vi "Main.vi"(11 "Module Admin":refnum<class "Delacor_lib_QMH_Module Admin.lvclass">) -> ()   [LabVIEW 2016, in "Impedance Acquisition.lvlib"]
doc: "This template is based off of the Queued Message Handler design pattern and the Queued Message Handler project template that ships with LabVIEW.\n\nThe main difference is that the queue is private to this module and communication between modules is performed via Broadcast and Request events.\n\nRequest events are wrapped in public API methods and are handled in the Event Handling Loop (EHL) of this VI. Any module can register for Broadcast events sent by this module. The EHL generates messages based on user interface actions.\n\nThe Message Handling Loop (MHL) processes messages generated by the EHL, or by other messages. The messages are string values, so new messages can be added easily to the Message Cases case structure in the MHL. Each message cluster can also provide an optional value for Message Data, which is a variant that can be converted to whatever message-specific data is required.\n_____\nBased on DQMH Project Template 6.1.0.94."
uses:
  Impedance Acquisition.lvlib
  <vilib>/Delacor/Delacor QMH/Libraries/Message Queue_class/Delacor_lib_QMH_Message Queue.lvclass
  Module Data--cluster.ctl
  <vilib>/Utility/miscctls.llb/LVPointTypeDef.ctl
  <vilib>/Utility/error.llb/Error Cluster From Error Code.vi
  <vilib>/ErrorRing/Error Ring.xnode
  <vilib>/Delacor/Delacor QMH/Libraries/Message Queue_class/Delacor_lib_QMH_Enqueue Message (Single).vi
  Stop Argument--cluster.ctl
  <vilib>/Delacor/Delacor QMH/Libraries/Module Admin_class/Delacor_lib_QMH_Module Admin.lvclass
  Settings Editor/Settings Editor.lvlib
  Acquisition/Reg_Map.ctl
  Acquisition/Acquisition.lvlib
  Acquisition/WiBCI16T_Status.ctl
  Acquisition/WiBCI16T_Data.ctl
  Start IMP Acq Argument--cluster.ctl
  Start GND LOOP Imp Argument--cluster.ctl
  Stop Imp Acq Argument--cluster.ctl
panel:
  out "error out":errorcluster
  out "Status":string
  in  "Simulate MHL Error":bool
  in  "Simulate EHL Error":bool
  # "Other QMH Modules communicate with this Module via its Public API (wrappers for its Request Events).\n\nThis Module communicates with other Modules via its Broadcast Events.\nAny module that wants to get these messages, just registers for this module's Broadcast events."
  # "This template is for the Delacor Modified Queued Message Handler design pattern.\n\nSee the block diagram for more information on how to use this template."
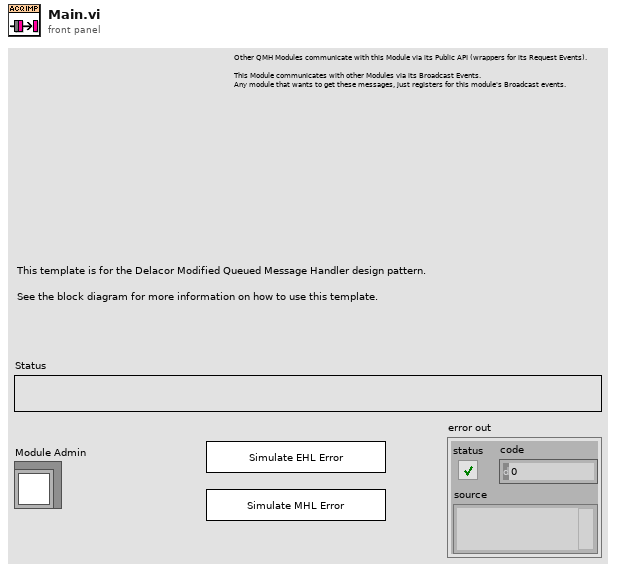
[diagram p1: front panel]
types:
  T1 = typedef "Impedance Acquisition.lvlib/Request Events--cluster.ctl" = cluster{"Stop Module":refnum<user-event>, "Show Panel":refnum<user-event>, "Hide Panel":refnum<user-event>, "Get Module Execution Status":refnum<user-event>, "Show Diagram":refnum<user-event>, "Start IMP Acq":refnum<user-event>, "Start GND LOOP Imp":refnum<user-event>, "Stop Imp Acq":refnum<user-event>}
  T2 = typedef "Settings Editor.lvlib/Broadcast Events--cluster.ctl" = cluster{"Module Did Init":refnum<user-event>, "Status Updated":refnum<user-event>, "Error Reported":refnum<user-event>, "Module Did Stop":refnum<user-event>, "Update Module Execution Status":refnum<user-event>, "Application Settings Updated":refnum<user-event>}
  T3 = typedef "Impedance Acquisition.lvlib/Module Data--cluster.ctl" = cluster{"Status":string, "WiBCI16T Data":T4}
  T4 = typedef "Acquisition.lvlib/WiBCI16T_Data.ctl" = cluster{"EEG Ch 1":dbl, "EEG Ch 2":dbl, "EEG Ch 3":dbl, "EEG Ch 4":dbl, "EEG Ch 5":dbl, "EEG Ch 6":dbl, "EEG Ch 7":dbl, "EEG Ch 8":dbl, "EEG Ch 9":dbl, "EEG Ch 10":dbl, "EEG Ch 11":dbl, "EEG Ch 12":dbl, "EEG Ch 13":dbl, "EEG Ch 14":dbl, "EEG Ch 15":dbl, "EEG Ch 16":dbl, "X-Accel":i16, "Y-Accel":i16, "Z-Accel":i16, "X-Gyro":i16, "Y-Gyro":i16, "Z-Gyro":i16, "Timer":u32, "Packet ID":u32, "HW Trig1":u8, "SW Trig1":i8, "HW Trig2":u8, "SW Trig2":i8, "WiBCI Status":T5, "Reg Map":T6}
  T5 = typedef "Acquisition.lvlib/WiBCI16T_Status.ctl" = cluster{"Mode Byte":u8, "Ch Config":u8, "Ch Ref Map":u16, "Ch Enable Map":u16, "Temperature":sgl, "Battery":u8, "Version":string}
  T6 = typedef "Acquisition.lvlib/Reg_Map.ctl" = cluster{"ADS1":u8[], "ADS2":u8[]}
  T7 = enum32{"invalid lock state", "Not Locked", "Locked (No Password)", "Password-protected"}
  T8 = typedef "Impedance Acquisition.lvlib/Stop Argument--cluster.ctl" = cluster{"Origin":string, "Exit via Stop Module Req?":bool, "Wait for Module to stop?":bool}
  T9 = typedef "Impedance Acquisition.lvlib/Start IMP Acq Argument--cluster.ctl" = cluster{"En Ch":u16, "Ref Ch":u16}
  T10 = typedef "Impedance Acquisition.lvlib/Start GND LOOP Imp Argument--cluster.ctl" = cluster{"En Ch":u16, "Ref Ch":u16}
  T11 = typedef "Impedance Acquisition.lvlib/Stop Imp Acq Argument--cluster.ctl" = cluster{"Boolean":bool}
  T12 = typedef "LVPointTypeDef.ctl" = cluster{"Horizontal":i16, "Vertical":i16}
  T13 = enum32{"Invalid", "Standard", "Closed", "Hidden", "Minimized", "Maximized"}
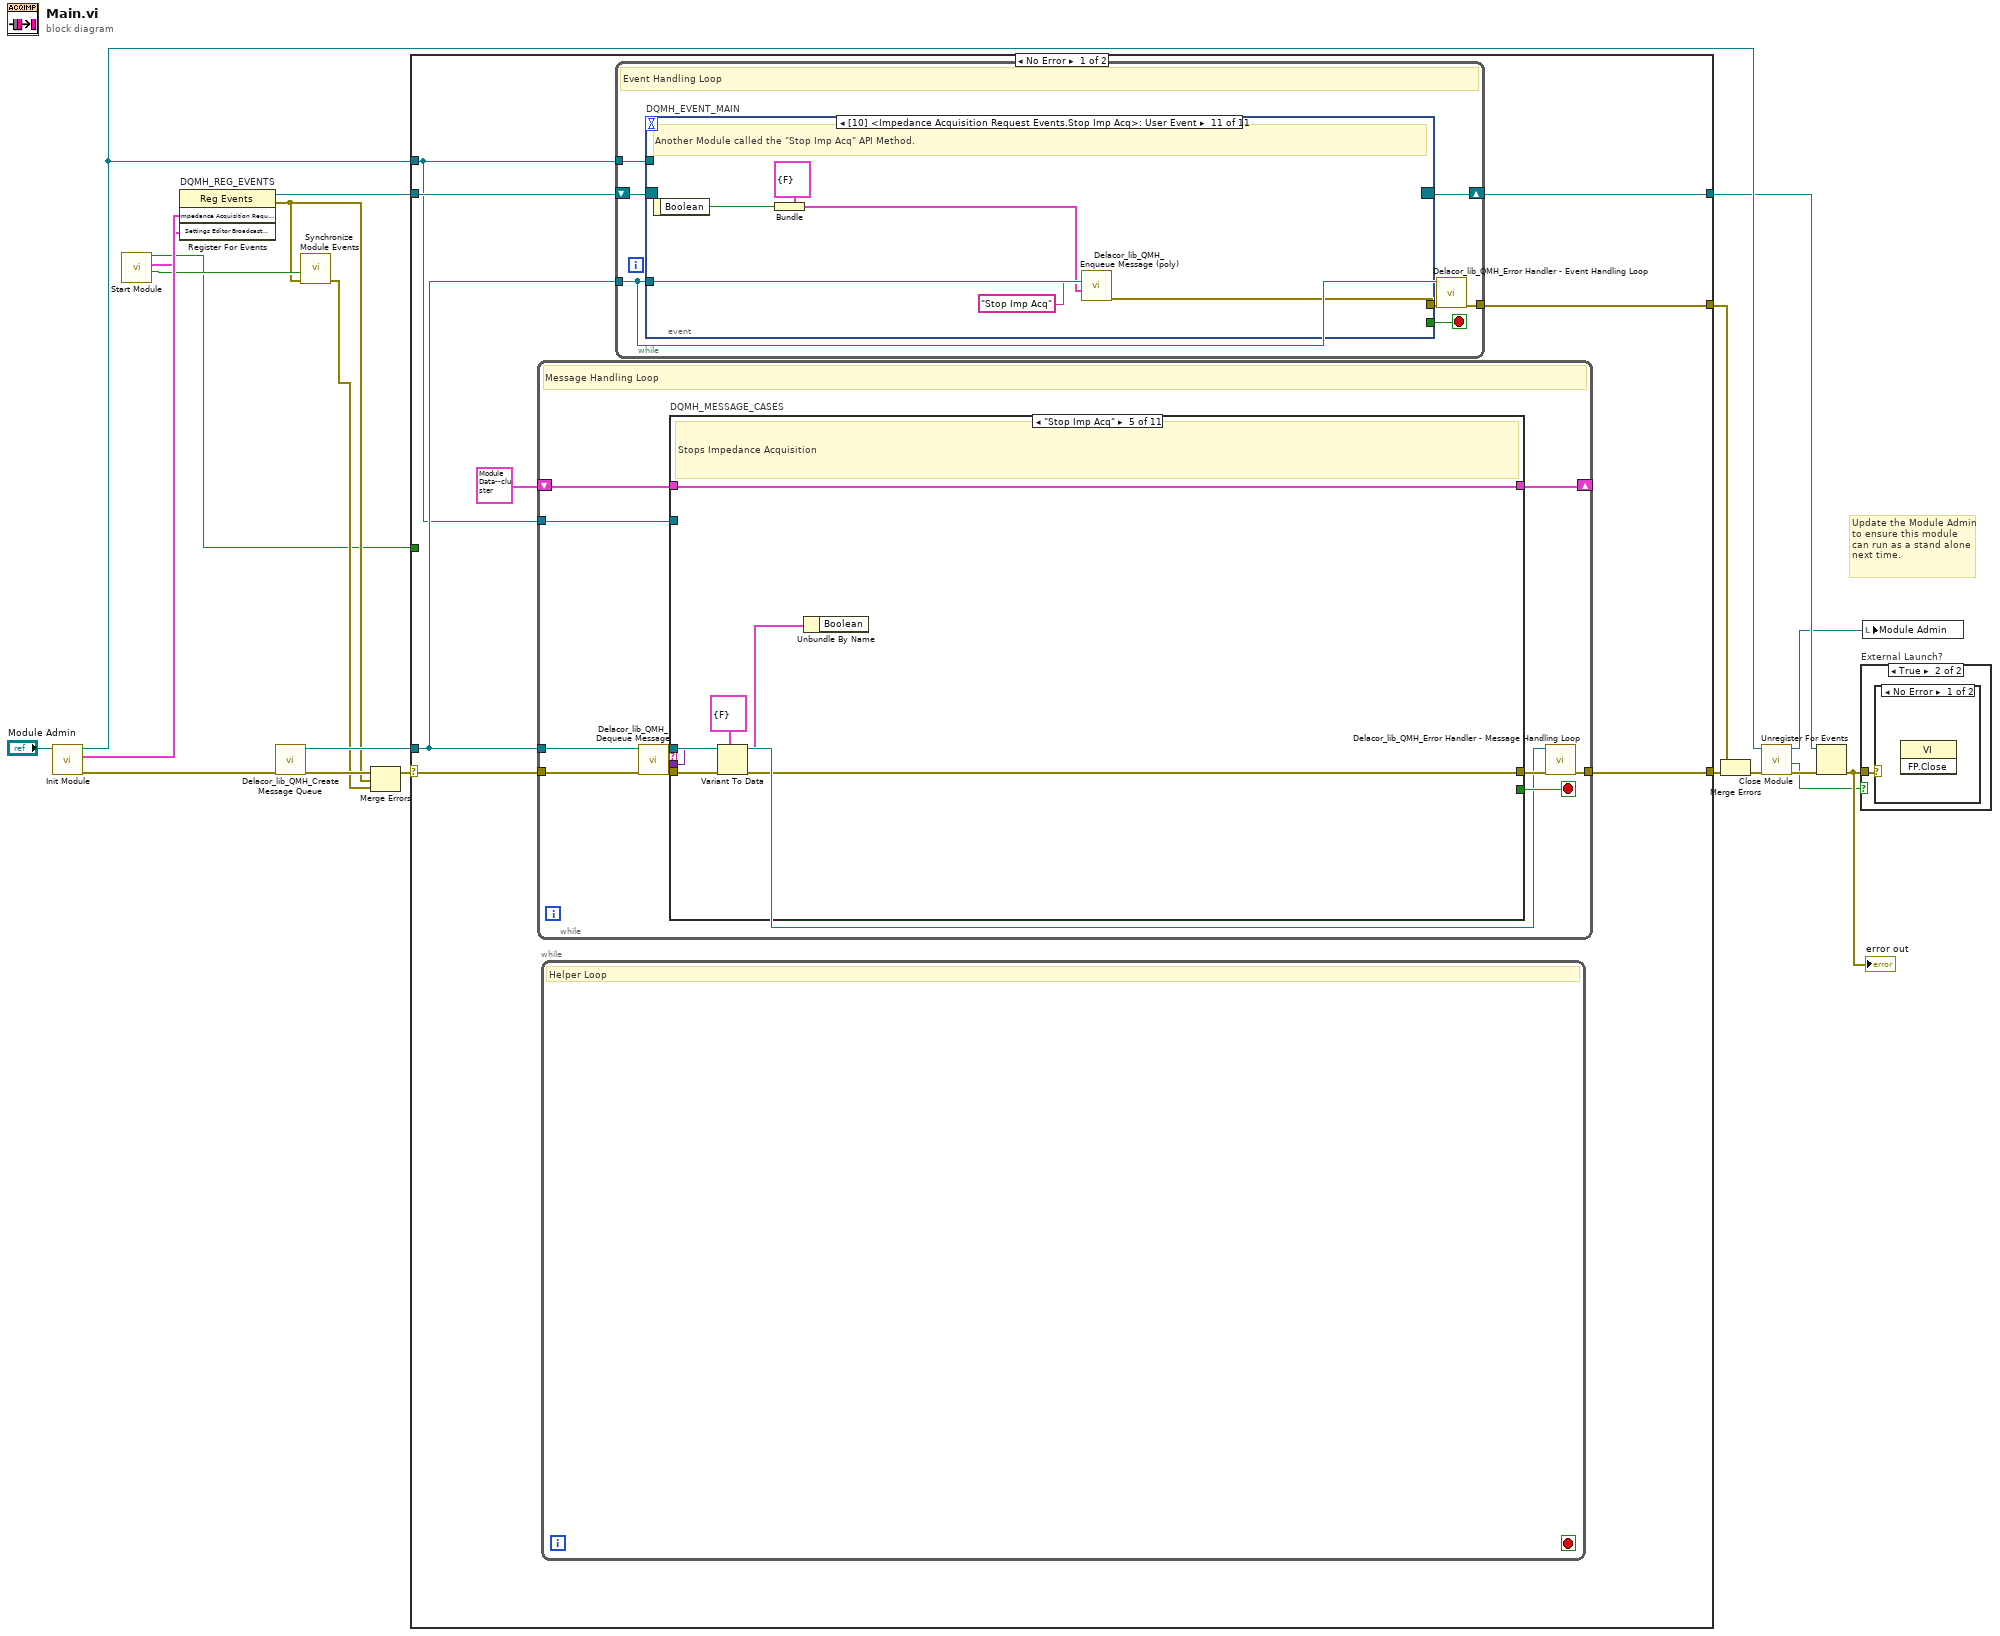
[diagram p0: block diagram]
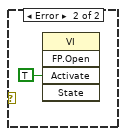
[diagram p3: hidden frame]
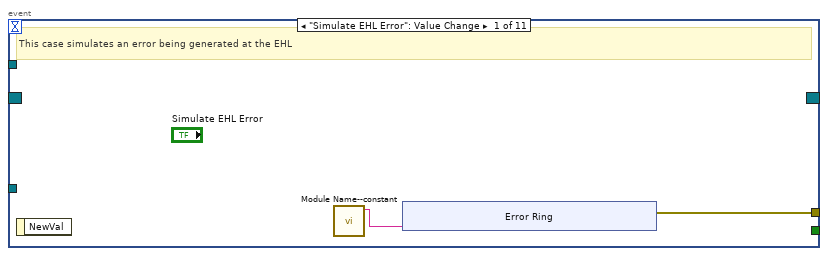
[diagram p4: hidden frame]
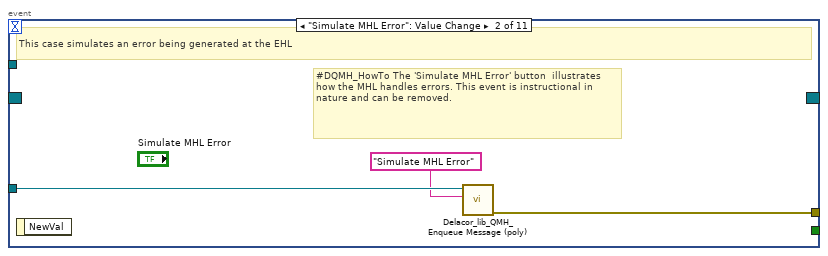
[diagram p5: hidden frame]
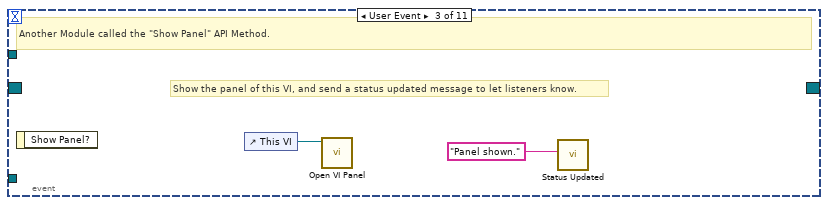
[diagram p6: hidden frame]
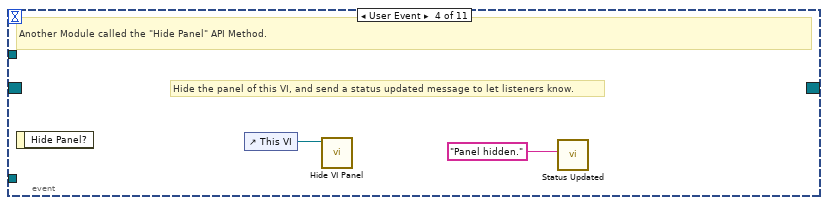
[diagram p7: hidden frame]
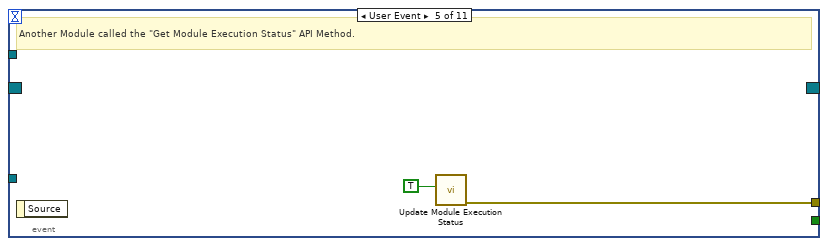
[diagram p8: hidden frame]
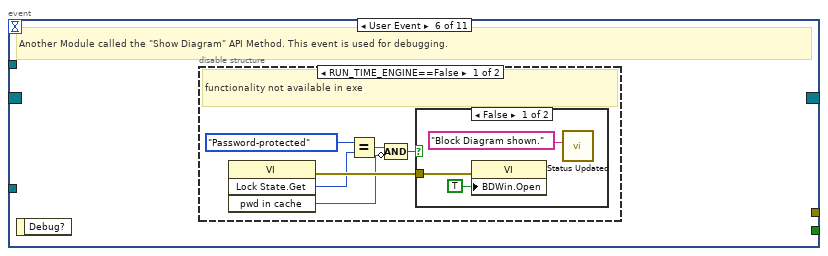
[diagram p9: hidden frame]
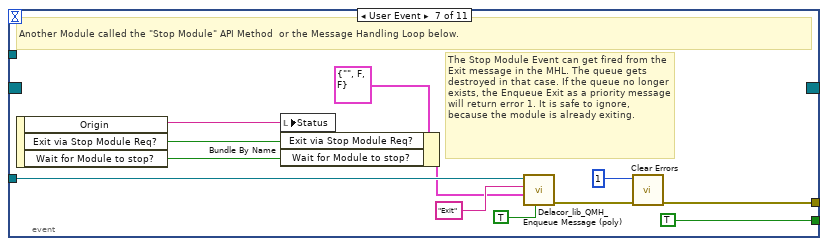
[diagram p12: hidden frame]
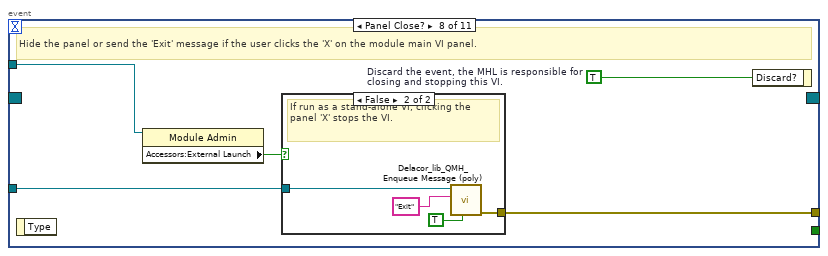
[diagram p13: hidden frame]
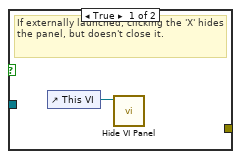
[diagram p14: hidden frame]
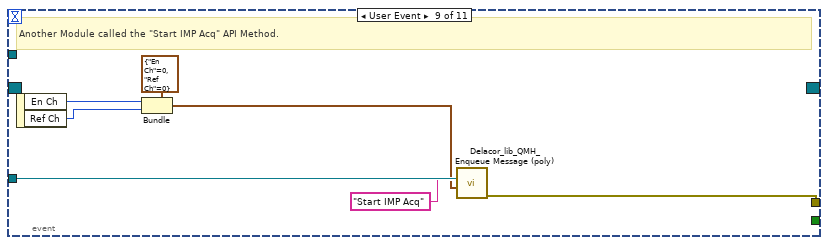
[diagram p15: hidden frame]
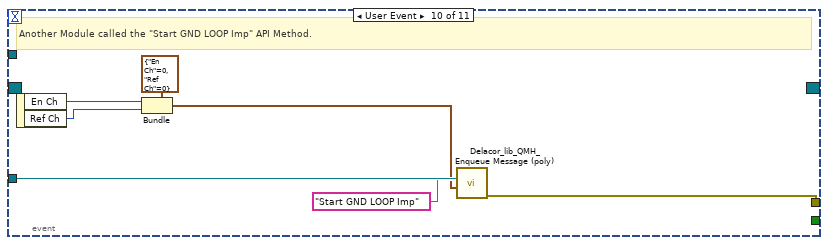
[diagram p16: hidden frame]
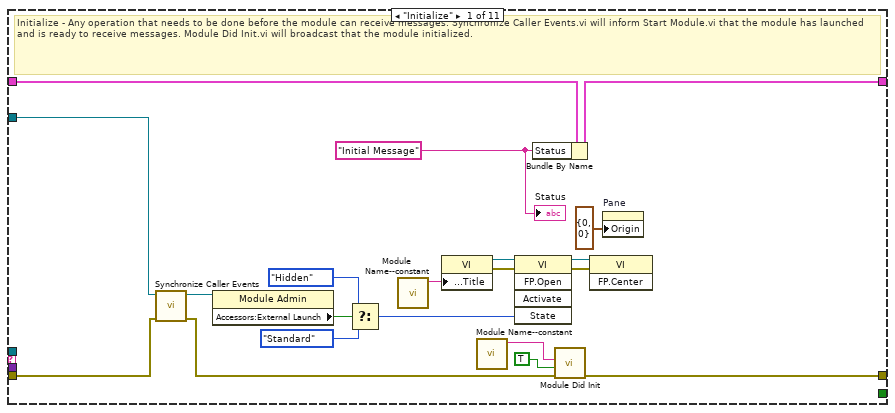
[diagram p17: hidden frame]
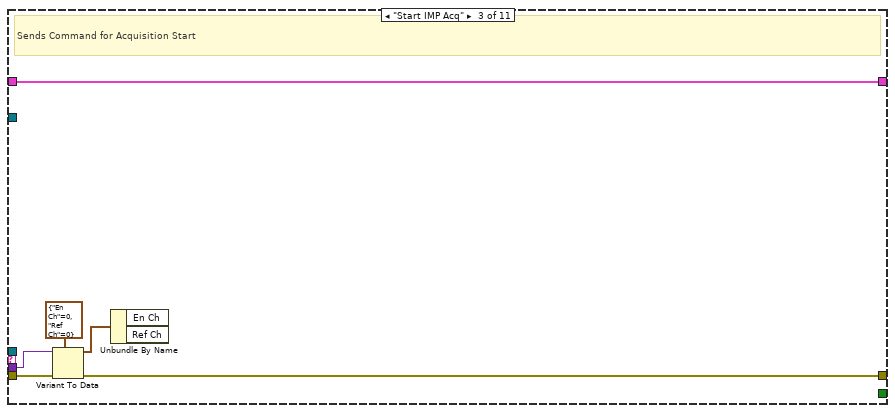
[diagram p19: hidden frame]
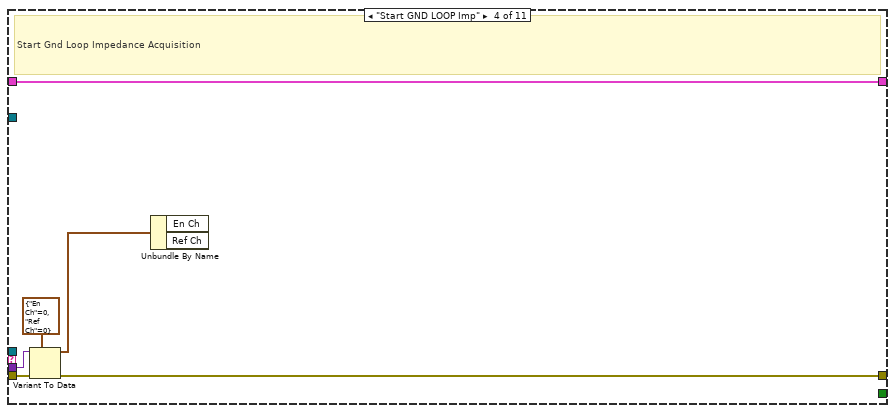
[diagram p20: hidden frame]
diagram:
  # "Update the Module Admin to ensure this module can run as a stand alone next time."
  n1 = call "Init Module.vi"("Singleton Module Admin in"="Module Admin") -> ("error out"=w20:errorcluster, "Impedance Acquisition Request Events"=w10:T1, "Singleton Module Admin out"=w13:refnum<class "Delacor_lib_QMH_Module Admin.lvclass">)  [unwired: 8 in]
  n2 = call "Start Module.vi"() -> ("Wait for Event Sync?"=w4:bool, "Settings Editor Broadcast Events"=w5:T2, "Module Was Already Running?"=w1:bool)  [unwired: 8 in, 1 out]
  n3 = register-events "DQMH_REG_EVENTS"(w10, w5) -> (reference out=w11:refnum<event-registration>, error out=w3:errorcluster)  [unwired: 2 in]
  n4 = call <vilib>:"Delacor_lib_QMH_Create Message Queue.vi"("error in"=w20) -> ("error out"=w15:errorcluster, "Message Queue"=w9:refnum<class "Delacor_lib_QMH_Message Queue.lvclass">)  [unwired: 9 in]
  n5 = call "Synchronize Module Events.vi"("error in (no error)"=w3, "Wait for Event Sync?"=w4) -> ("error out"=w2:errorcluster)  [unwired: 9 in]
  n6 = Merge Errors(w15, w3, w2) -> (w14:errorcluster)
  n7 = case shown="No Error" w14 {
    selector: w14 -> [w27 w222]
    tunnel: [w29 w221] -> w21
    tunnel: [w26 w227] -> w12
    tunnel: w11 -> [w24 w227]
    tunnel: w9 -> [w23 w220]
    tunnel: [w28 _] -> w18
    tunnel: w13 -> [w22 w223]
    tunnel: w1 -> [_ _]
    frame No Error {
      n8 = while {
        tunnel: w23 -> [w108]
        shift-right: [w112] -> _
        shift-left: T3 {"Status"="", "WiBCI16T Data"={"EEG Ch 1"=0.0, "EEG Ch 2"=0.0, "EEG Ch 3"=0.0, "EEG Ch 4"=0.0, "EEG Ch 5"=0.0, "EEG Ch 6"=0.0, "EEG Ch 7"=0.0, "EEG Ch 8"=0.0, "EEG Ch 9"=0.0, "EEG Ch 10"=0.0, "EEG Ch 11"=0.0, "EEG Ch 12"=0.0, "EEG Ch 13"=0.0, "EEG Ch 14"=0.0, "EEG Ch 15"=0.0, "EEG Ch 16"=0.0, "X-Accel"=0, "Y-Accel"=0, "Z-Accel"=0, "X-Gyro"=0, "Y-Gyro"=0, "Z-Gyro"=0, "Timer"=0, "Packet ID"=0, "HW Trig1"=0, "SW Trig1"=0, "HW Trig2"=0, "SW Trig2"=0, "WiBCI Status"={"Mode Byte"=0, "Ch Config"=0, "Ch Ref Map"=0, "Ch Enable Map"=0, "Temperature"=0.0, "Battery"=0, "Version"=""}, "Reg Map"={"ADS1"=[], "ADS2"=[]}}} ("Data Cluster") -> [w113]
        tunnel: w27 -> [w116]
        tunnel: [w114] -> w29
        tunnel: w22 -> [w106]
        stop <- w111 stop-if-true
        # "Message Handling Loop"
        n9 = call-dynamic "Delacor_lib_QMH_Dequeue Message.vi"("error in"=w116, "Message Queue in"=w108) -> ("error out"=w115:errorcluster, "Message Data"=w109:variant, "Message"=w110:string, "Message Queue out"=w107:refnum<class "Delacor_lib_QMH_Message Queue.lvclass">)  [unwired: 6 in]
        n10 = case "DQMH_MESSAGE_CASES" shown="\"Stop Imp Acq\"" w110 {
          selector: w110 -> [_ _ _ _ _ _ _ _ _ _ w207]
          tunnel: w107 -> [_ _ _ _ _ _ _ _ w177 w199 _]
          tunnel: w115 -> [w135 w139 w145 w151 w157 w160 w162 w167 w184 w205 w209]
          tunnel: [w133 w139 w143 w149 w155 w159 w162 w166 w180 w202 w210] -> w117
          tunnel: w113 -> [w124 w138 w144 w150 w156 w158 w161 w164 w179 w198 w208]
          tunnel: [w123 w138 w144 w150 w156 w158 w161 w164 w179 w198 w208] -> w112
          tunnel: [_ _ _ _ _ _ _ _ _ w197 _] -> w111
          tunnel: w109 -> [_ _ w142 w148 w154 _ _ _ w178 w196 _]
          tunnel: w106 -> [w125 _ _ _ _ _ _ _ w176 w191 _]
          frame "Initialize" {
            w119 = "Initial Message" ("Initial Message")
            # "Initialize - Any operation that needs to be done before the module can receive messages. Synchronize Caller Events.vi will inform Start Module.vi that the module has launched and is ready to receive messages. Module Did Init.vi will broadcast that the module initialized."
            n11 = call "Synchronize Caller Events.vi"("error in (no error)"=w135, "Singleton Module Admin in"=w125) -> ("error out"=w134:errorcluster, "Singleton Module Admin out"=w120:refnum<class "Delacor_lib_QMH_Module Admin.lvclass">)  [unwired: 8 in]
            n12 = property class="Module Admin"(reference=w120) -> ("Accessors:External Launch"=w129:bool)  [unwired: 1 in, 2 out]
            n13 = Select(t=T13."Hidden" ("State"), s=w129, f=T13."Standard" ("State")) -> (s? t:f=w126:T13)
            n14 = call "Module Name--constant.vi"() -> ("Module Name"=w132:string)  [unwired: 11 in]
            n15 = property class="VI"("Front Panel.Title"=w132) -> (reference out=w131:refnum<vi>, error out=w137:errorcluster)  [unwired: 2 in]
            n16 = call "Module Name--constant.vi"() -> ("Module Name"=w121:string)  [unwired: 11 in]
            n17 = invoke class="VI" method="FP.Open"(reference=w131, error in=w137, "State"=w126) -> (reference out=w130:refnum<vi>, error out=w136:errorcluster)  [unwired: 2 in, 3 out]
            n18 = Bundle By Name(cluster=w124, "Status"=w119) -> (w123:T3)
            n19 = call "Module Did Init.vi"("error in (no error)"=w134, "Initialized?"=TRUE, "Origin"=w121) -> ("error out"=w133:errorcluster)  [unwired: 8 in]
            n20 = invoke class="VI" method="FP.Center"(reference=w130, error in=w136) -> ()  [unwired: 1 in, 3 out]
            n21 = property on="Pane" class="Pane"("Origin"=T12 {"Horizontal"=0, "Vertical"=0}) -> ()  [unwired: 2 in, 2 out]
            "Status" <- w119
          }
          frame "---Module Specific---" {
            # "Separator -- The following cases handle messages specific to this Module."
          }
          frame "Start IMP Acq" {
            # "Sends Command for Acquisition Start"
            n22 = Variant To Data(error in=w145, type=T9 {"En Ch"=0, "Ref Ch"=0} ("Start IMP Acq Argument"), Variant=w142) -> (data=w140:T9, error out=w143:errorcluster)
            n23 = Unbundle By Name(w140) -> ()  [unwired: 2 out]
          }
          frame "Start GND LOOP Imp" {
            # "Start Gnd Loop Impedance Acquisition"
            n24 = Variant To Data(error in=w151, type=T10 {"En Ch"=0, "Ref Ch"=0} ("Start GND LOOP Imp Argument"), Variant=w148) -> (data=w146:T10, error out=w149:errorcluster)
            n25 = Unbundle By Name(w146) -> ()  [unwired: 2 out]
          }
          frame "Stop Imp Acq" {
            # "Stops Impedance Acquisition"
            n26 = Variant To Data(error in=w157, type=T11 {"Boolean"=FALSE} ("Stop Imp Acq Argument"), Variant=w154) -> (data=w152:T11, error out=w155:errorcluster)
            n27 = Unbundle By Name(w152) -> ()  [unwired: 1 out]
          }
          frame "---Copy This Frame---" {
            # "Duplicate this frame when creating new messages.  Change this comment in the duplicated frame to describe this message."
            n28 = Merge Errors(w160) -> (w159:errorcluster)
          }
          frame "---Exit and Error Handling---" {
            # "Separator - The following cases handle errors and exit messages."
          }
          frame "Simulate MHL Error" {
            # "#DQMH_HowTo The 'Simulate MHL Error' button  illustrates how the MHL handles errors. This event is instructional in nature and can be removed."
            # "Simulate an error occurring at the MHL"
            n29 = call "Module Name--constant.vi"() -> ("Module Name"=w163:string)  [unwired: 11 in]
            n30 = xnode "Error Ring"("parameter 0"=w163) -> ("error out"=w165:errorcluster)
            n31 = Merge Errors(w167, w165) -> (w166:errorcluster)
          }
          frame "Error" {
            # "#CodeRecommended - If you ever change the name of this \"Error\" message, you'll need to update the name in the Check Loop Error.vi as well."
            # "#CodeRecommended - If the module is running in standalone mode (External Launch = FALSE), this code will pop up an error dialog and call the 'Exit' message if an error occurs. Add more fine-grained error handling here."
            # "Error - Check the error message data and respond accordingly. This message is sent by the \"Error Handler\" VIs at the end of each loop in this application."
            n32 = property class="Module Admin"(reference=w176) -> ("Accessors:External Launch"=w175:bool)  [unwired: 1 in, 2 out]
            n33 = Variant To Data(error in=w184, type=errorcluster {"status"=FALSE, "code"=0, "source"=""} ("error constant"), Variant=w178) -> (data=w185:errorcluster, error out=w182:errorcluster)
            n34 = call "Error Reported.vi"("Error"=w185) -> ()  [unwired: 10 in, 1 out]
            n35 = case shown="False" w175 {
              tunnel: [w190 _] -> w181
              tunnel: w177 -> [w188 _]
              tunnel: w185 -> [w189 _]
              frame False {
                # "If the module is running standalone, then pop up an error dialog and call the \"Exit\" message."
                n36 = call <vilib>:"Simple Error Handler.vi"("error in (no error)"=w189) -> ()  [unwired: 4 in, 5 out]
                n37 = call-poly <vilib>:"Delacor_lib_QMH_Enqueue Message (poly).vi"("Priority Message? (F)"=TRUE, "Message"="Exit", "Message Queue in"=w188) -> ("error out"=w190:errorcluster)  [unwired: 7 in, 1 out]
              }
              frame True {
                # "If the module was launched externally, calling the Error Reported broadcast VI is the only action performed by the \"Error\" message. The module's caller can then process the error appropriately."
              }
            }
            n38 = Merge Errors(w182, w181) -> (w180:errorcluster)
            n39 = local write "error out"(w180) -> ()
          }
          frame "Exit" {
            w195 = 91  # 91: not all Exit messages will have an argument
            w197 = TRUE  # Stop the VI
            # "Release the message queue reference"
            # "#CodeNeeded - Add any required cleanup code here"
            # "Exit - Exit the application."
            n40 = Variant To Data(error in=w205, type=T8 {"Origin"="", "Exit via Stop Module Req?"=FALSE, "Wait for Module to stop?"=FALSE} ("Stop Argument"), Variant=w196) -> (data=w193:T8, error out=w201:errorcluster)
            n41 = call <vilib>:"Clear Errors.vi"("error in (no error)"=w201, "specific error code to clear (0: all)"=w195) -> ("error out"=w204:errorcluster)  [unwired: 4 in, 1 out]
            n42 = control-ref of="This VI"() -> (w192:refnum<vi>)
            n43 = call-dynamic "Delacor_lib_QMH_Release Message Queue.vi"("error in"=w204, "Message Queue"=w199) -> ("error out"=w203:errorcluster)  [unwired: 9 in]
            n44 = call "Handle Exit.vi"("Stop Argument"=w193, "Admin in"=w191, "VI reference"=w192) -> ("error out"=w200:errorcluster)  [unwired: 7 in, 1 out]
            n45 = Merge Errors(w203, w200) -> (w202:errorcluster)
          }
          frame Default {
            # "'Default' case only runs if there is a message that isn't defined in any of the other cases.  Output a programming error."
            n46 = call "Module Name--constant.vi"() -> ("Module Name"=w206:string)  [unwired: 11 in]
            n47 = xnode "Error Ring"("parameter 0"=w207, "parameter 1"=w206) -> ("error out"=w211:errorcluster)
            n48 = Merge Errors(w209, w211) -> (w210:errorcluster)
          }
        }
        n49 = call-dynamic "Delacor_lib_QMH_Error Handler - Message Handling Loop.vi"("error in"=w117, "Message Queue in"=w107) -> ("dup error in"=w114:errorcluster)  [unwired: 8 in, 1 out]
      }
      n50 = while {
        stop <- _ stop-if-true
        # "Helper Loop"
      }
      n51 = while {
        tunnel: w23 -> [w30]
        shift-right: [w33] -> w26
        shift-left: w24 -> [w34]
        tunnel: [w35] -> w28
        tunnel: w22 -> [w31]
        stop <- w32 stop-if-true
        # "Event Handling Loop"
        n52 = event "DQMH_EVENT_MAIN" shown="[10] <Impedance Acquisition Request Events.Stop Imp Acq>: User Event" {
          selector: w34 -> [_ _ _ _ _ _ _ _ _ _ _]
          dyn-events: [_ _ _ _ _ _ _ _ _ _ _] -> w33
          timeout: _ -> [_ _ _ _ _ _ _ _ _ _ _]
          tunnel: [_ _ _ _ _ _ TRUE ("Discard?") _ _ _ _] -> w32
          tunnel: w30 -> [_ w47 _ _ _ _ w71 w78 w92 w99 w105]
          tunnel: [w38 w48 _ _ w54 _ w74 w80 w86 w93 w100] -> w36
          tunnel: w31 -> [_ _ _ _ _ _ _ w77 _ _ _]
          event "Simulate EHL Error": Value Change {
            # "This case simulates an error being generated at the EHL"
            n53 = event-data() -> ()  [unwired: 1 in, 1 out]
            n54 = call "Module Name--constant.vi"() -> ("Module Name"=w37:string)  [unwired: 11 in]
            n55 = xnode "Error Ring"("parameter 0"=w37) -> ("error out"=w38:errorcluster)
          }
          event "Simulate MHL Error": Value Change {
            # "#DQMH_HowTo The 'Simulate MHL Error' button  illustrates how the MHL handles errors. This event is instructional in nature and can be removed."
            # "This case simulates an error being generated at the EHL"
            n56 = event-data() -> ()  [unwired: 1 in, 1 out]
            n57 = call-poly <vilib>:"Delacor_lib_QMH_Enqueue Message (poly).vi"("Message"="Simulate MHL Error", "Message Queue in"=w47) -> ("error out"=w48:errorcluster)  [unwired: 8 in, 1 out]
          }
          event User Event {
            # "Show the panel of this VI, and send a status updated message to let listeners know."
            # "Another Module called the \"Show Panel\" API Method."
            n58 = event-data() -> ()  [unwired: 1 in, 1 out]
            n59 = control-ref of="This VI"() -> (w50:refnum<vi>)
            n60 = call "Open VI Panel.vi"("VI"=w50) -> ()  [unwired: 10 in, 1 out]
            n61 = call "Status Updated.vi"("Status"="Panel shown." ("format string")) -> ()  [unwired: 10 in, 1 out]
          }
          event User Event {
            # "Hide the panel of this VI, and send a status updated message to let listeners know."
            # "Another Module called the \"Hide Panel\" API Method."
            n62 = event-data() -> ()  [unwired: 1 in, 1 out]
            n63 = control-ref of="This VI"() -> (w52:refnum<vi>)
            n64 = call "Hide VI Panel.vi"("VI"=w52) -> ()  [unwired: 10 in, 1 out]
            n65 = call "Status Updated.vi"("Status"="Panel hidden." ("format string")) -> ()  [unwired: 10 in, 1 out]
          }
          event User Event {
            # "Another Module called the \"Get Module Execution Status\" API Method."
            n66 = event-data() -> ()  [unwired: 1 in, 1 out]
            n67 = call "Update Module Execution Status.vi"("Running?"=TRUE) -> ("error out"=w54:errorcluster)  [unwired: 10 in]
          }
          event User Event {
            # "Another Module called the \"Show Diagram\" API Method. This event is used for debugging."
            n68 = event-data() -> ()  [unwired: 1 in, 1 out]
            n69 = disable-structure shown="RUN_TIME_ENGINE==False" {
              frame condition #0 (active) {
                # "functionality not available in exe"
                n70 = invoke class="VI" method="Lock State.Get"() -> (error out=w60:errorcluster, "Get Lock State"=w59:T7, "pwd in cache"=w56:bool)  [unwired: 4 in, 1 out]
                n71 = Equal?(x=T7."Password-protected", y=w59) -> (x = y?=w57:bool)
                n72 = Compound Arithmetic op=AND(w57, invert w56) -> (w55:bool)
                n73 = case shown="False" w55 {
                  tunnel: w60 -> [w63 _]
                  frame False {
                    n74 = property class="VI"(error in=w63, "BDWin.Open"=TRUE ("Block Diagram Window:Open")) -> ()  [unwired: 1 in, 2 out]
                    n75 = call "Status Updated.vi"("Status"="Block Diagram shown." ("format string")) -> ()  [unwired: 10 in, 1 out]
                  }
                  frame True {
                    # "Password-protected VI, and the password is not in the cache. Do not show the diagram."
                  }
                }
              }
              frame condition #1 {
              }
            }
          }
          event User Event {
            # "The Stop Module Event can get fired from the Exit message in the MHL. The queue gets destroyed in that case. If the queue no longer exists, the Enqueue Exit as a priority message will return error 1. It is safe to ignore, because the module is already exiting."
            # "Another Module called the \"Stop Module\" API Method  or the Message Handling Loop below."
            n76 = event-data() -> ("Origin"=w70:string, "Exit via Stop Module Req?"=w66:bool, "Wait for Module to stop?"=w65:bool)  [unwired: 1 in]
            n77 = local write "Status"(w70) -> ()
            n78 = Bundle By Name(cluster=T8 {"Origin"="", "Exit via Stop Module Req?"=FALSE, "Wait for Module to stop?"=FALSE} ("Stop Argument"), "Exit via Stop Module Req?"=w66, "Wait for Module to stop?"=w65) -> (w64:T8)
            n79 = call-poly <vilib>:"Delacor_lib_QMH_Enqueue Message (poly).vi"("Priority Message? (F)"=TRUE, "Message Data"=w64, "Message"="Exit", "Message Queue in"=w71) -> ("error out"=w75:errorcluster)  [unwired: 6 in, 1 out]
            n80 = call <vilib>:"Clear Errors.vi"("error in (no error)"=w75, "specific error code to clear (0: all)"=1) -> ("error out"=w74:errorcluster)  [unwired: 4 in, 1 out]
          }
          event Panel Close? {
            w79 = TRUE  # Discard the event, the MHL is responsible for closing and stopping this VI.
            # "Hide the panel or send the 'Exit' message if the user clicks the 'X' on the module main VI panel."
            n81 = event-data() -> ()  [unwired: 1 in, 1 out]
            n82 = property class="Module Admin"(reference=w77) -> ("Accessors:External Launch"=w76:bool)  [unwired: 1 in, 2 out]
            n83 = case shown="False" w76 {
              tunnel: w78 -> [_ w84]
              tunnel: [_ w85] -> w80
              frame True {
                # "If externally launched, clicking the 'X' hides the panel, but doesn't close it."
                n84 = control-ref of="This VI"() -> (w81:refnum<vi>)
                n85 = call "Hide VI Panel.vi"("VI"=w81) -> ()  [unwired: 10 in, 1 out]
              }
              frame False {
                # "If run as a stand-alone VI, clicking the panel 'X' stops the VI."
                n86 = call-poly <vilib>:"Delacor_lib_QMH_Enqueue Message (poly).vi"("Priority Message? (F)"=TRUE, "Message"="Exit", "Message Queue in"=w84) -> ("error out"=w85:errorcluster)  [unwired: 7 in, 1 out]
              }
            }
            n87 = event-data("Discard?"=w79) -> ()  [unwired: 1 in, 1 out]
          }
          event User Event {
            # "Another Module called the \"Start IMP Acq\" API Method."
            n88 = event-data() -> ("En Ch"=w88:u16, "Ref Ch"=w87:u16)  [unwired: 1 in]
            n89 = Bundle(cluster=T9 {"En Ch"=0, "Ref Ch"=0} ("Start IMP Acq Argument"), "En Ch"=w88, "Ref Ch"=w87) -> (w89:T9)
            n90 = call-poly <vilib>:"Delacor_lib_QMH_Enqueue Message (poly).vi"("Message Data"=w89, "Message"="Start IMP Acq", "Message Queue in"=w92) -> ("error out"=w86:errorcluster)  [unwired: 7 in, 1 out]
          }
          event User Event {
            # "Another Module called the \"Start GND LOOP Imp\" API Method."
            n91 = event-data() -> ("En Ch"=w95:u16, "Ref Ch"=w94:u16)  [unwired: 1 in]
            n92 = Bundle(cluster=T10 {"En Ch"=0, "Ref Ch"=0} ("Start GND LOOP Imp Argument"), "En Ch"=w95, "Ref Ch"=w94) -> (w96:T10)
            n93 = call-poly <vilib>:"Delacor_lib_QMH_Enqueue Message (poly).vi"("Message Data"=w96, "Message"="Start GND LOOP Imp", "Message Queue in"=w99) -> ("error out"=w93:errorcluster)  [unwired: 7 in, 1 out]
          }
          event User Event {
            # "Another Module called the \"Stop Imp Acq\" API Method."
            n94 = event-data() -> ("Boolean"=w101:bool)  [unwired: 1 in]
            n95 = Bundle(cluster=T11 {"Boolean"=FALSE} ("Stop Imp Acq Argument"), "Boolean"=w101) -> (w102:T11)
            n96 = call-poly <vilib>:"Delacor_lib_QMH_Enqueue Message (poly).vi"("Message Data"=w102, "Message"="Stop Imp Acq", "Message Queue in"=w105) -> ("error out"=w100:errorcluster)  [unwired: 7 in, 1 out]
          }
        }
        n97 = call-dynamic "Delacor_lib_QMH_Error Handler - Event Handling Loop.vi"("error in"=w36, "Message Queue in"=w30) -> ("dup error in"=w35:errorcluster)  [unwired: 8 in, 1 out]
      }
    }
    frame Error {
      # "Synchronize Caller Events.vi will inform Start Module.vi that the module has launched and will let the code calling Start Module.vi register for broadcasts and would permit the caller receive the broadcast that an error occurred at launch time."
      n98 = call-dynamic "Delacor_lib_QMH_Release Message Queue.vi"("error in"=w222, "Message Queue"=w220) -> ("error out"=w221:errorcluster)  [unwired: 9 in]
      n99 = call "Synchronize Caller Events.vi"("Singleton Module Admin in"=w223) -> ("error out"=w228:errorcluster)  [unwired: 9 in, 1 out]
      n100 = call "Module Name--constant.vi"() -> ("Module Name"=w226:string)  [unwired: 11 in]
      n101 = Format Into String(format string="An error occurred during initialization. %s is no longer running.", w226) -> (resulting string=w224:string)  [unwired: 2 in, 1 out]
      n102 = Merge Errors(w221, w228) -> (w229:errorcluster)
      n103 = call "Error Reported.vi"("Additional Information"=w224, "Error"=w229) -> ()  [unwired: 9 in, 1 out]
    }
  }
  n104 = Merge Errors(w18, w21) -> (w17:errorcluster)
  n105 = call "Close Module.vi"("error in (no error)"=w17, "Module Admin in"=w13) -> ("error out"=w19:errorcluster, "External Launch"=w6:bool, "Module Admin out"=w7:refnum<class "Delacor_lib_QMH_Module Admin.lvclass">)  [unwired: 7 in]
  n106 = Unregister For Events(event registration refnum=w12, error in=w19) -> (error out=w16:errorcluster)
  "error out" <- w16
  n107 = case "External Launch?" shown="True" w6 {
    tunnel: w16 -> [_ w230]
    frame False {
    }
    frame True {
      n108 = case shown="No Error" w230 {
        frame No Error {
          n109 = invoke class="VI" method="FP.Close"() -> ()  [unwired: 3 in, 3 out]
        }
        frame Error {
          n110 = invoke class="VI" method="FP.Open"("Activate"=TRUE ("Activate?")) -> ()  [unwired: 4 in, 5 out]
        }
      }
    }
  }
  n111 = local write "Module Admin"(w7) -> ()
